vi "Get_UTC.vi"(1 "UTC numeric":dbl format="%<%H:%M:%S%0u>t") -> (0 "UTC string":string)   [LabVIEW 2010]
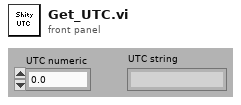
[diagram p1: front panel]
types:
  T1 = typedef "LVDateTimeRec.ctl" = cluster{"fractional second":dbl, "second":i32, "minute":i32, "hour":i32, "day of month":i32, "month":i32, "year":i32, "day of week":i32, "day of year":i32, "DST":i32}
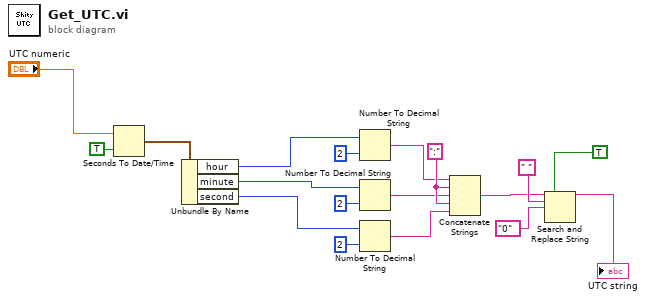
[diagram p0: block diagram]
diagram:
  w14 = ":"
  n1 = Seconds To Date/Time(time stamp (now)="UTC numeric", to UTC (F)=TRUE) -> (date time rec=w2:T1)
  n2 = Unbundle By Name(w2) -> ("hour"=w7:i32, "minute"=w6:i32, "second"=w5:i32)
  n3 = Number To Decimal String(number=w7, width (-)=i16 2) -> (decimal integer string=w11:string)
  n4 = Number To Decimal String(number=w6, width (-)=i16 2) -> (decimal integer string=w12:string)
  n5 = Number To Decimal String(number=w5, width (-)=i16 2) -> (decimal integer string=w13:string)
  n6 = Concatenate Strings(w11, w14, w12, w14, w13) -> (w15:string)
  n7 = Search and Replace String(replace all?=TRUE ("replace all? (F)"), input string=w15, search string=" ", replace string="0" ("replace string (\"\")")) -> (result string=→"UTC string":string)  [unwired: 4 in, 3 out]
